vi "SRV_Prompt for Single Line Entry.vi"(0 "Prompt":string="Enter text below.", 5 "Default Entry String (\"\")":string, 7 "True String (OK)":string="OK", 9 "False String (Cancel)":string="Cancel") -> (6 "Entered String":string, 8 "True/OK":bool, 10 "Canceled":bool)   [LabVIEW 2009]
doc: "This VI is use to prompt the user for a single line string entry.\n\nAuthor: Mike Schultz"
panel:
  in  "Cancel":bool
  in  "OK":bool
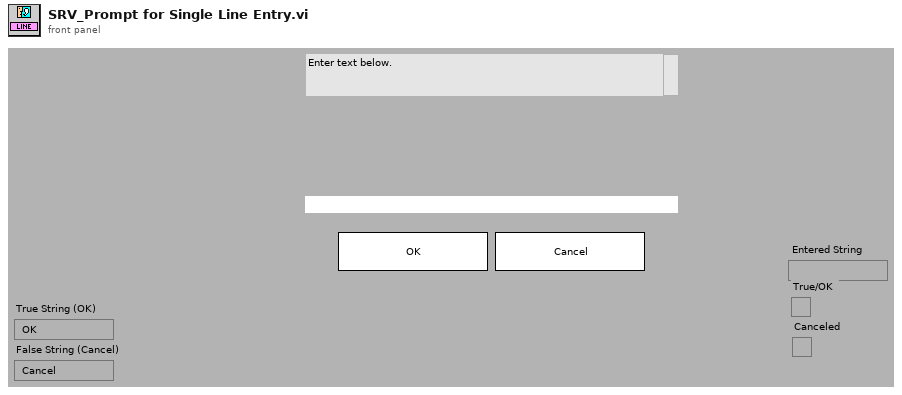
[diagram p1: front panel]
types:
  T1 = enum8{"Enabled", "Disabled", "Disabled and Grayed Out"}
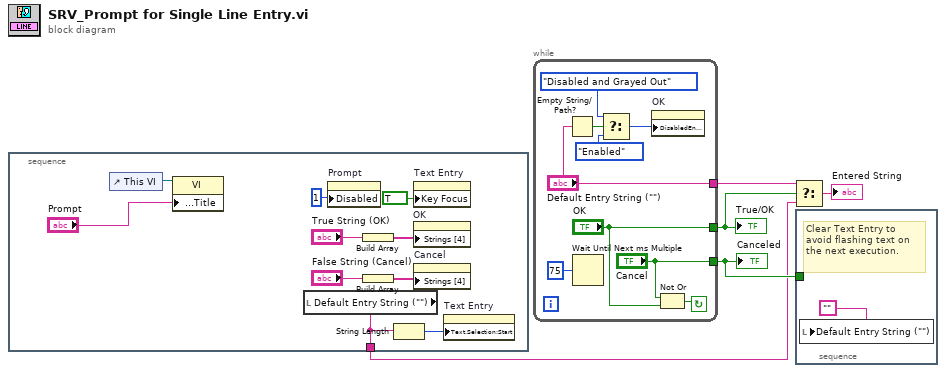
[diagram p0: block diagram]
diagram:
  n1 = stacked-sequence {
    tunnel: [w9] -> w1
    frame #0 {
      n2 = control-ref of="This VI"() -> (w6:refnum<vi>)
      n3 = property class="VI"(reference=w6, "Front Panel Window:Title"="Prompt") -> ()  [unwired: 1 in, 2 out]
      n4 = local read "Default Entry String (\"\")"() -> (w9:string)
      n5 = property on="Prompt" class="String"("Disabled"=u8 1) -> ()  [unwired: 2 in, 2 out]
      n6 = Build Array("True String (OK)") -> (w14:string[])
      n7 = Build Array("False String (Cancel)") -> (w15:string[])
      n8 = String Length(string=w9) -> (length=w10:i32)
      n9 = property on="Text Entry" class="String"("Key Focus"=TRUE) -> ()  [unwired: 2 in, 2 out]
      n10 = property on="OK" class="Boolean"("Strings [4]"=w14) -> ()  [unwired: 2 in, 2 out]
      n11 = property on="Cancel" class="Boolean"("Strings [4]"=w15) -> ()  [unwired: 2 in, 2 out]
      n12 = property on="Text Entry" class="String"("Text.Selection:Start"=w10) -> ()  [unwired: 2 in, 2 out]
    }
  }
  n13 = while {
    tunnel: ["Default Entry String (\"\")"] -> w4
    tunnel: ["Cancel"] -> w2
    tunnel: ["OK"] -> w5
    stop <- w24 continue-if-true
    n14 = Empty String/Path?(string/path="Default Entry String (\"\")") -> (empty?=w19:bool)
    n15 = Wait Until Next ms Multiple(millisecond multiple=u32 75) -> ()  [unwired: 1 out]
    n16 = Select(t=T1."Disabled and Grayed Out" ("Disabled"), s=w19, f=T1."Enabled" ("Disabled")) -> (s? t:f=w16:T1)
    n17 = property on="OK" class="Boolean"("DisabledEnum"=w16) -> ()  [unwired: 2 in, 2 out]
    n18 = Not Or(1:"OK", 2:"Cancel") -> (0:w24:bool)
  }
  "Canceled" <- w2
  "True/OK" <- w5
  n19 = Select(t=w4, s=w5, f=w1) -> (s? t:f=→"Entered String":string)
  n20 = stacked-sequence {
    tunnel: w2 -> [_]
    frame #0 {
      # "Clear Text Entry to avoid flashing text on the next execution."
      n21 = local write "Default Entry String (\"\")"("") -> ()
    }
  }
